vi "tm_getframe_wview.vi"(8 "error in (no error)":errorcluster {"code" format="%.0x"}, 9 "Frame Index":i32=-1, 10 "Buffer Info":T1, 11 "Handle in":u32) -> (0 "error out":errorcluster {"code" format="%.0x"}, 1 "Data B":u16[][](array[numeric]), 2 "Data A":u16[][](array[numeric]), 3 "Handle out":u32, 4 "Electron Info":cluster{"coefficient":sgl, "offset":sgl})   [LabVIEW 2023]
uses:
  tmcamcon.dll
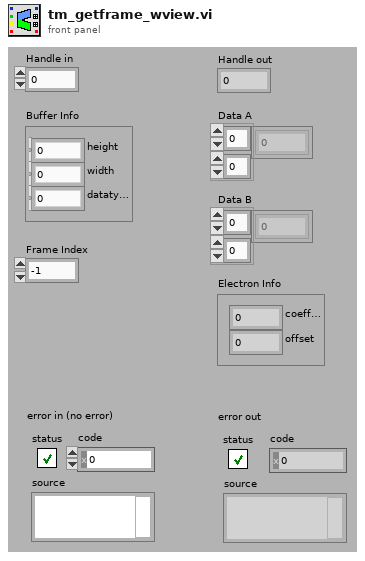
[diagram p1: front panel]
types:
  T1 = cluster{"height":u32, "width":u32, "datatype":u32}
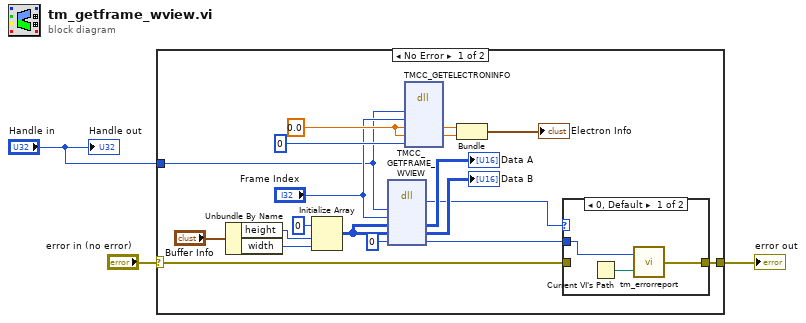
[diagram p0: block diagram]
diagram:
  n1 = case shown="No Error" "error in (no error)" {
    selector: "error in (no error)" -> [w21 w27]
    tunnel: [w20 w27] -> w2
    tunnel: "Handle in" -> [w7 _]
    frame No Error {
      w14 = sgl 0.0 ("C")
      n2 = Unbundle By Name("Buffer Info") -> ("height"=w19:u32, "width"=w18:u32)
      n3 = Initialize Array(u16 0 ("element"), w19, w18) -> (w12:u16[][])
      n4 = dll-call lib="tmcamcon.dll" fn="TMCC_GETFRAME_WVIEW"("index"=w7, "frameindex"="Frame Index", "imgarray1"=w12, "imgarray2"=w12, "Erval"=0) -> ("return type"=w6:u32, "imgarray1"=→"Data A":u16[][], "imgarray2"=→"Data B":u16[][], "Erval"=w5:i32)  [unwired: 5 in, 2 out]
      n5 = dll-call lib="tmcamcon.dll" fn="TMCC_GETELECTRONINFO"("index"=w7, "frame"="Frame Index", "C"=w14, "O"=w14, "Erval"=0) -> ("C"=w16:sgl, "O"=w15:sgl)  [unwired: 7 in, 2 out]
      n6 = Bundle("C"=w16, "O"=w15) -> (→"Electron Info":cluster{"C":sgl, "O":sgl})  [unwired: 1 in]
      n7 = case shown="0, Default" w6 {
        tunnel: w21 -> [_ w26]
        tunnel: [w24 w26] -> w20
        tunnel: w5 -> [w23 _]
        frame 0, Default {
          n8 = Current VI's Path() -> (path=w25:path)
          n9 = call "tm_errorreport.vi"("Source"=w25, "Error"=w23) -> ("error out"=w24:errorcluster)
        }
        frame 1 {
        }
      }
    }
    frame Error {
    }
  }
  "error out" <- w2
  "Handle out" <- "Handle in"
